vi "test-trapezoid-profile-execute.vi"() -> (3 "Test Passed":bool)   [LabVIEW 2019]
uses:
  <vilib>/Rock Robotics/WPI/ThirdParty/JAS_Junk/TrajLib/LinearFilter_ResetToValue.vi
  <vilib>/Rock Robotics/WPI/ThirdParty/JAS_Junk/TrajLib/LinearFilter_Calculate.vi
  <vilib>/Rock Robotics/WPI/ThirdParty/JAS_Junk/TrajLib/TrapProfile_Calculate.vi
  <vilib>/Rock Robotics/WPI/ThirdParty/JAS_Junk/TrajLib/TrapProfile_New.vi
  <vilib>/Rock Robotics/WPI/ThirdParty/JAS_Junk/TrajLib/TrapProfile_TotalTime.vi
  <vilib>/Rock Robotics/WPI/ThirdParty/JAS_Junk/TrajLib/TrapProfConstraint_New.vi
  <vilib>/Rock Robotics/WPI/ThirdParty/JAS_Junk/TrajLib/TrapProfState_New.vi
  <vilib>/Rock Robotics/WPI/ThirdParty/JAS_Junk/TrajLib/TrapProfile_IsFinished.vi
  <vilib>/Rock Robotics/WPI/ThirdParty/JAS_Junk/TrajLib/TrapProfile_Direct.vi
  <vilib>/Rock Robotics/WPI/ThirdParty/JAS_Junk/TrajLib/TrapProfile_ShouldFlipAcceleration.vi
  <vilib>/Rock Robotics/SystemInterfaces/NetworkCommunication/NetComm_UsageReport_report.vi
  <vilib>/Rock Robotics/WPI/ThirdParty/JAS_Junk/TrajLib/LinearFilter_MovingAverage.vi
  <vilib>/Rock Robotics/WPI/ThirdParty/JAS_Junk/TrajLib/LinearFilter_LowPassBW1.vi
  <vilib>/Rock Robotics/WPI/ThirdParty/JAS_Junk/TrajLib/LinearFilter_LowPassBW2.vi
  <vilib>/Rock Robotics/WPI/ThirdParty/JAS_Junk/TrajLib/LinearFilter_HighPassBW1.vi
  <vilib>/Rock Robotics/WPI/ThirdParty/JAS_Junk/TrajLib/LinearFilter_HighPassBW2.vi
  <vilib>/Rock Robotics/WPI/ThirdParty/JAS_Junk/TrajLib/Util_LibraryGlobals.vi
  <vilib>/Rock Robotics/WPI/ThirdParty/JAS_Junk/TrajLib/Trajectory_Library.lvlib
panel:
  out "ApproxEquals 2":bool
  out "ApproxEquals":bool
  out "LibUsage_ProfiledPID":i32 format="%20.0f"
  out "LibUsage_PIDController":i32 format="%20.0f"
  out "LibUsage_Odometry":i32 format="%20.0f"
  out "LibUsage_LinearFIlter":i32 format="%20.0f"
  out "LibUsage_TrapezoidProfile":i32 format="%20.0f"
  out "LibUsage_Kinematics":i32 format="%20.0f"
  out "ActVel":dbl
  out "ActAccel":dbl
  out "ElapsedTIme":dbl format="%20.6f"
  in  "Position\nGoal":dbl=2.0 format="%#_13g"
  out "EstTimeLeft":dbl format="%23.3f"
  out "VelocityDmd":dbl
  out "PositionDmd":dbl
  out "Waveform Chart":T1(graph)
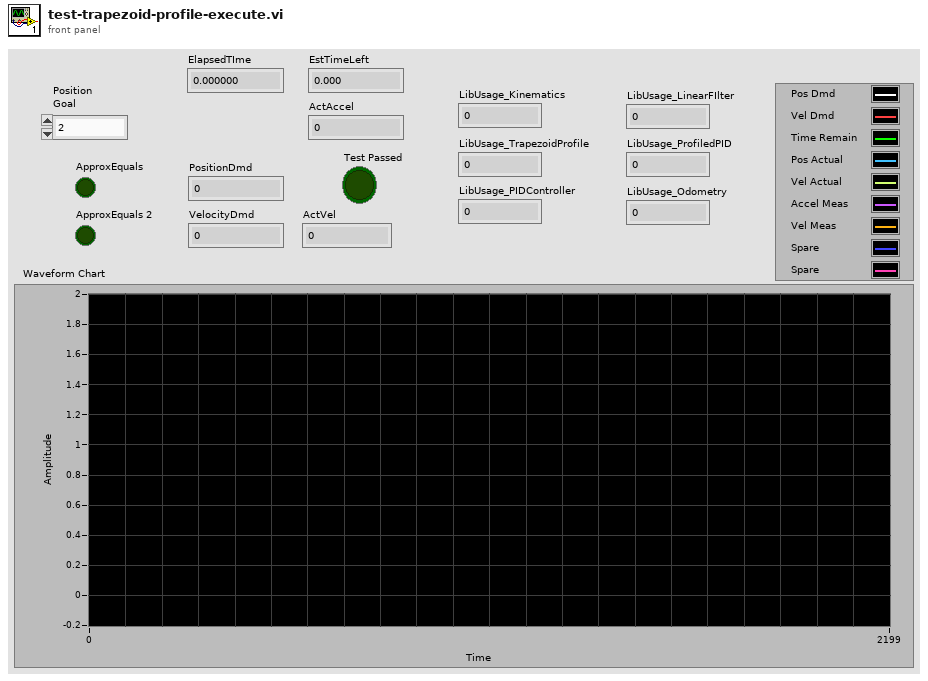
[diagram p1: front panel]
types:
  T1 = cluster{"PositionDmd":dbl, "VelocityDmd":dbl, "EstTimeLeft":dbl, "Output":dbl, "Output":dbl, dbl, dbl, dbl, dbl}
  T2 = enum16{"Moving Average", "Low Pass 1st Order Butterworth", "Low Pass 2nd Order Butterworth", "High Pass 1st Order Butterworth", "High Pass 2nd Order Butterworth"}
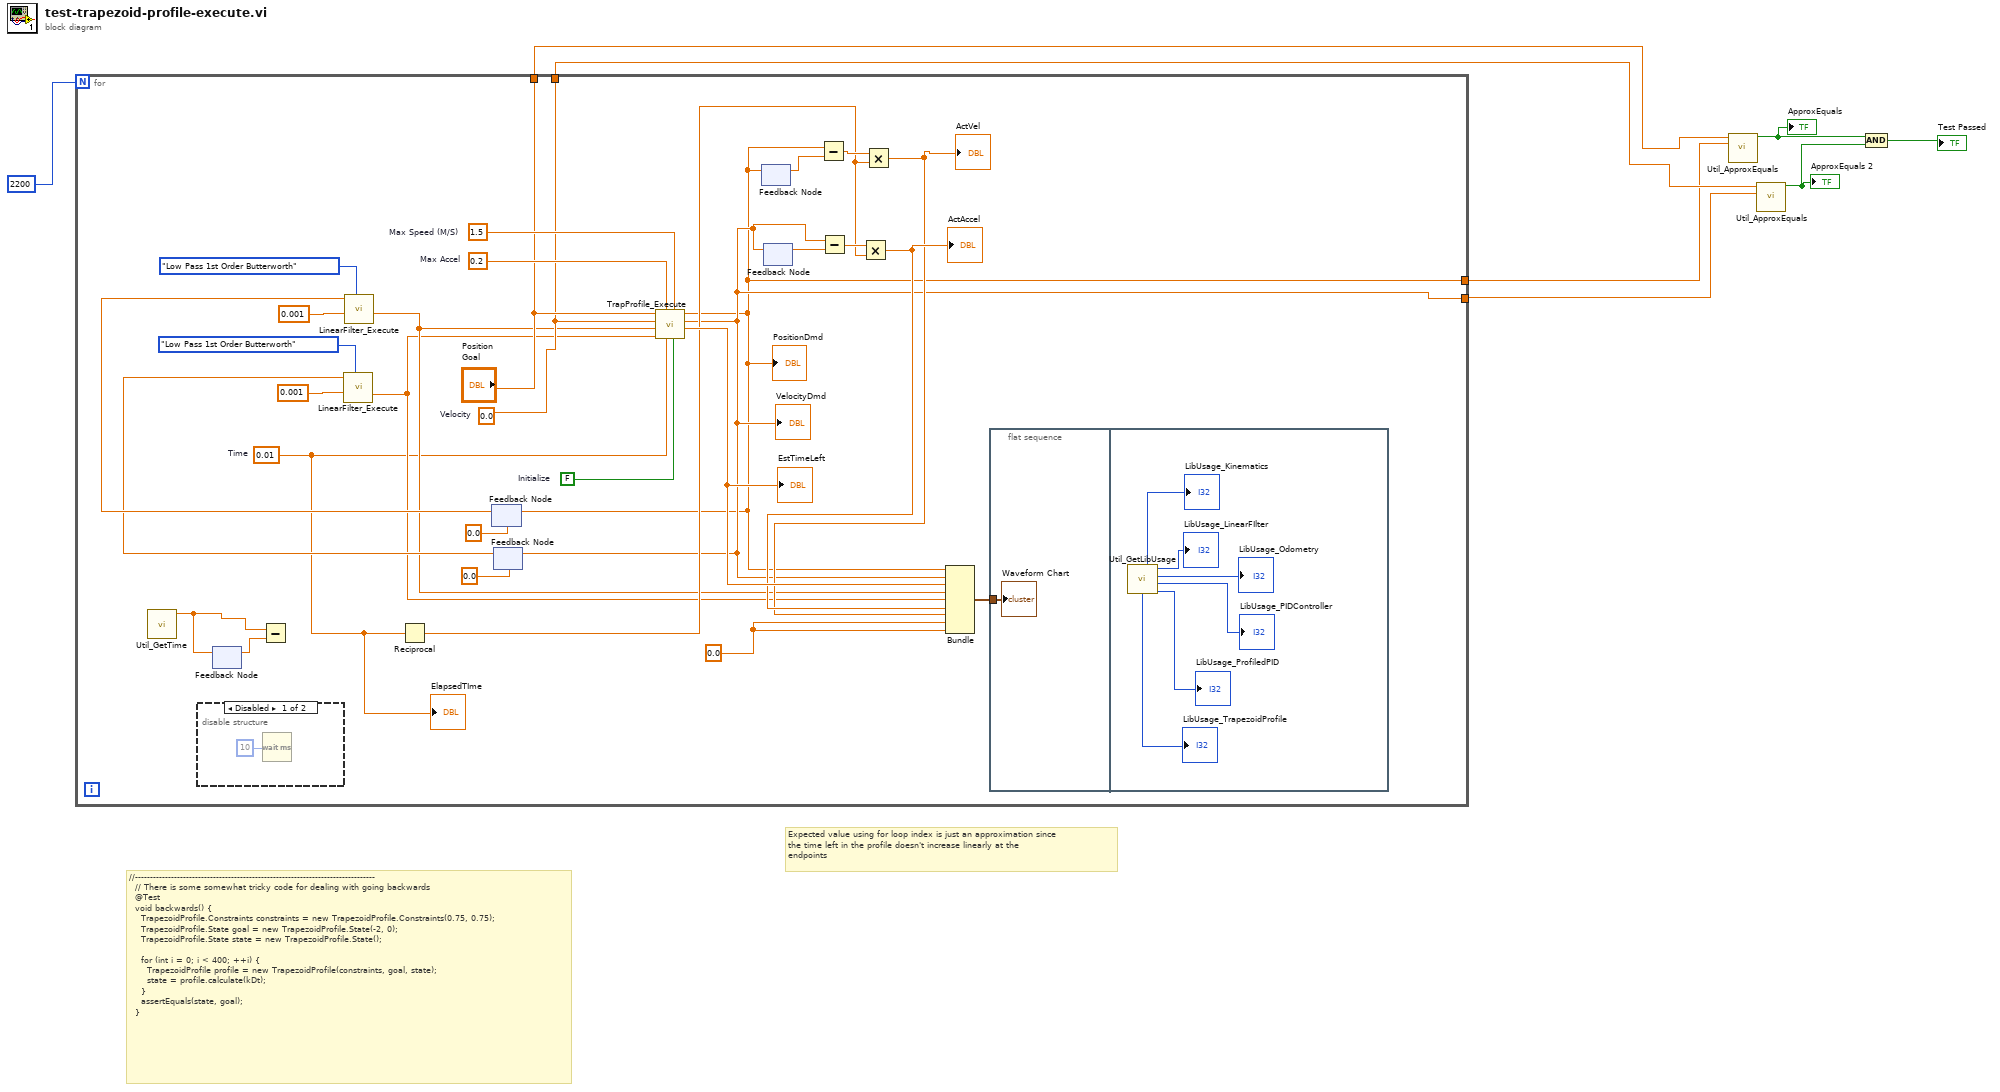
[diagram p0: block diagram]
diagram:
  # "Expected value using for loop index is just an approximation since\nthe time left in the profile doesn't increase linearly at the\nendpoints"
  # "//--------------------------------------------------------------------------------\n  // There is some somewhat tricky code for dealing with going backwards\n  @Test\n  void backwards() {\n    TrapezoidProfile.Constraints constraints = new TrapezoidProfile.Constraints(0.75, 0.75);\n    TrapezoidProfile.State goal = new TrapezoidProfile.State(-2, 0);\n    TrapezoidProfile.State state = new TrapezoidProfile.State();\n\n    for (int i = 0; i < 400; ++i) {\n      TrapezoidProfile profile = new TrapezoidProfile(constraints, goal, state);\n      state = profile.calculate(kDt);\n    }\n    assertEquals(state, goal);\n  }"
  n1 = for {
    N: 2200 -> [_]
    tunnel: ["Position\nGoal"] -> w4
    tunnel: [w13] -> w3
    tunnel: [w10] -> w2
    tunnel: [w16] -> w1
    w15 = FALSE  # Initialize
    w23 = 0.0
    w13 = 0.0  # Velocity
    w37 = 0.2  # Max Accel
    w38 = 1.5  # Max Speed (M/S)
    w9 = 0.01  # Time
    n2 = call <vilib>:"Util_GetTime.vi"() -> ("FPGA_Time_Seconds"=w26:dbl)  [unwired: 10 in, 1 out]
    n3 = disable-structure shown="Disabled" {
      frame Disabled {
        n4 = Wait (ms)(milliseconds to wait=u32 10) -> ()  [unwired: 1 out]
      }
      frame Enabled {
      }
    }
    n5 = feedback-in #1(w26) -> ()
    n6 = feedback #1() -> (w25:dbl)  [unwired: 1 in]
    n7 = Subtract(x=w26, y=w25) -> ()  [unwired: 1 out]
    n8 = Reciprocal(x=w9) -> (1/x=w17:dbl)
    n9 = feedback #2(0.0 ("PositionDmd")) -> (w35:dbl)
    n10 = call <vilib>:"LinearFilter_Execute.vi"("Filter Type"=T2."Low Pass 1st Order Butterworth", "TimeConstant"=0.001, "Input"=w35) -> ("Output"=w12:dbl)  [unwired: 7 in, 1 out]
    n11 = feedback #3(0.0 ("VelocityDmd")) -> (w31:dbl)
    n12 = call <vilib>:"LinearFilter_Execute.vi"("Filter Type"=T2."Low Pass 1st Order Butterworth", "TimeConstant"=0.001, "Input"=w31) -> ("Output"=w11:dbl)  [unwired: 7 in, 1 out]
    n13 = call <vilib>:"TrapProfile_Execute.vi"("Initialize"=w15, "Max Speed"=w38, "TimePeriod"=w9, "Max Accel"=w37, "CurrentVelocity"=w11, "CurrentPosition"=w12, "GoalVelocity"=w13, "GoalPosition"="Position\nGoal") -> ("EstTimeLeft"=w30:dbl, "VelocityDmd"=w16:dbl, "PositionDmd"=w10:dbl)  [unwired: 1 out]
    "PositionDmd" <- w10
    "VelocityDmd" <- w16
    "EstTimeLeft" <- w30
    n14 = feedback-in #2(w10) -> ()
    n15 = feedback-in #3(w16) -> ()
    n16 = feedback #4() -> (w22:dbl)  [unwired: 1 in]
    n17 = feedback-in #4(w10) -> ()
    n18 = feedback #5() -> (w24:dbl)  [unwired: 1 in]
    n19 = feedback-in #5(w16) -> ()
    n20 = Subtract(x=w10, y=w22) -> (x-y=w19:dbl)
    n21 = Subtract(x=w16, y=w24) -> (x-y=w18:dbl)
    n22 = Multiply(x=w18, y=w17) -> (x*y=w21:dbl)
    "ActAccel" <- w21
    n23 = Multiply(x=w19, y=w17) -> (x*y=w20:dbl)
    "ActVel" <- w20
    n24 = Bundle("PositionDmd"=w10, "VelocityDmd"=w16, "EstTimeLeft"=w30, "Output"=w12, "Output"=w11, w21, w20, w23, w23) -> (w29:T1)  [unwired: 1 in]
    n25 = flat-sequence {
      tunnel: w29 -> [w40]
      frame #0 {
        "Waveform Chart" <- w40
      }
      frame #1 {
        n26 = call <vilib>:"Util_GetLibUsage.vi"() -> ("LibUsage_ProfiledPID"=→"LibUsage_ProfiledPID":i32, "LibUsage_PIDController"=→"LibUsage_PIDController":i32, "LibUsage_Odometry"=→"LibUsage_Odometry":i32, "LibUsage_LinearFIlter"=→"LibUsage_LinearFIlter":i32, "LibUsage_TrapezoidProfile"=→"LibUsage_TrapezoidProfile":i32, "LibUsage_Kinematics"=→"LibUsage_Kinematics":i32)  [unwired: 6 in]
      }
    }
    "ElapsedTIme" <- w9
  }
  n27 = call <vilib>:"Util_ApproxEquals.vi"("Value 2"=w2, "Value 1"=w4) -> ("ApproxEquals"=w6:bool)  [unwired: 9 in]
  "ApproxEquals" <- w6
  n28 = call <vilib>:"Util_ApproxEquals.vi"("Value 2"=w1, "Value 1"=w3) -> ("ApproxEquals"=w5:bool)  [unwired: 9 in]
  "ApproxEquals 2" <- w5
  n29 = And(x=w6, y=w5) -> (x .and. y?=→"Test Passed":bool)
